vi "Get DBECU Reference.vi"(8 "error in (no error)":errorcluster, 10 "Alias":string, 11 "Device Item Ref in":T1 format="%.0x") -> (0 "error out":errorcluster, 1 "empty?":bool, 2 "XNET ECU":refnum<k21>, 3 "Device Item Ref out":T1 format="%.0x", 5 "XNET Cluster":refnum<k21>)   [LabVIEW 2018, in "CAN Gateway System Explorer.lvlib"]
uses:
  CAN Gateway System Explorer.lvlib
  <vilib>/NI Veristand/Custom Device API/Custom Device Item Ref.ctl
  Shared/Constants.vi
  <vilib>/NI Veristand/Custom Device API/Get Item Property (String).vi
  <resource>/objmgr/xnet.rc
  <vilib>/NI Veristand/Custom Device API/Custom Device API.lvlib
  Shared/CAN Gateway Shared.lvlib
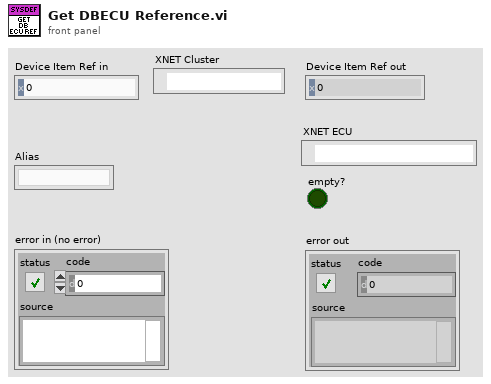
[diagram p1: front panel]
types:
  T1 = typedef "Custom Device API.lvlib/Custom Device Item Ref.ctl" = u64
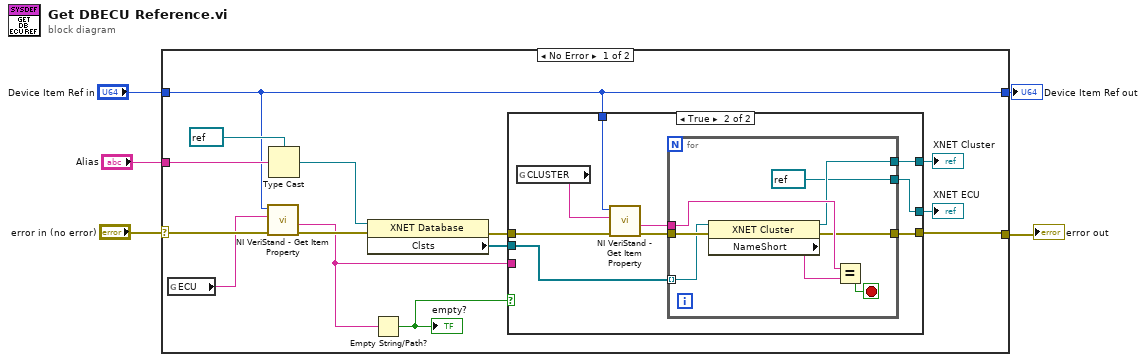
[diagram p0: block diagram]
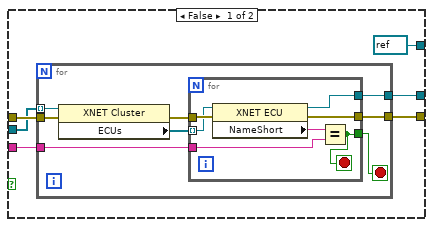
[diagram p2: hidden frame]
diagram:
  n1 = case shown="No Error" "error in (no error)" {
    selector: "error in (no error)" -> [w13 w59]
    tunnel: "Device Item Ref in" -> [w6 w58]
    tunnel: [w6 w58] -> w3
    tunnel: [w14 w59] -> w2
    tunnel: "Alias" -> [w19 _]
    frame No Error {
      n2 = global read "Constants.vi" "ECU"() -> (w12:string)
      n3 = call-poly <vilib>:"NI VeriStand - Get Item Property.vi"("error in (no error)"=w13, "Property Name"=w12, "Item Ref in"=w6) -> ("error out"=w11:errorcluster, "Value"=w9:string)  [unwired: 5 in, 2 out]
      n4 = Type Cast(type=refnum<k21> refnum ("XNET Database"), x=w19) -> (*(type *) &x=w17:refnum<k21>)
      n5 = property class="XNET Database"(reference=w17, error in=w11) -> (error out=w16:errorcluster, "Clsts"=w15:refnum<k21>[])  [unwired: 1 out]
      n6 = Empty String/Path?(string/path=w9) -> (empty?=w8:bool)
      "empty?" <- w8
      n7 = case shown="True" w8 {
        tunnel: w16 -> [w25 w48]
        tunnel: w15 -> [w24 w46]
        tunnel: [w23 w42] -> w14
        tunnel: [w22 w43] -> w10
        tunnel: w9 -> [w21 _]
        tunnel: [refnum<k21> refnum ("XNET Cluster") w44] -> w7
        tunnel: w6 -> [_ w41]
        frame False {
          n8 = for {
            tunnel: w25 -> [w33]
            tunnel: w24 -> [w32] mode=indexing
            tunnel: [w29] -> w23
            tunnel: w21 -> [w28]
            tunnel: [w27] -> w22
            stop <- w26 stop-if-true
            n9 = property class="XNET Cluster"(reference=w32, error in=w33) -> (error out=w30:errorcluster, "ECUs"=w31:refnum<k21>[])  [unwired: 1 out]
            n10 = for {
              tunnel: w31 -> [w39] mode=indexing
              tunnel: w30 -> [w40]
              tunnel: [w38] -> w29
              tunnel: w28 -> [w36]
              tunnel: [w35] -> w27
              tunnel: [w34] -> w26
              stop <- w34 stop-if-true
              n11 = property class="XNET ECU"(reference=w39, error in=w40) -> (reference out=w35:refnum<k21>, error out=w38:errorcluster, "NameShort"=w37:string)
              n12 = Equal?(x=w37, y=w36) -> (x = y?=w34:bool)
            }
          }
        }
        frame True {
          n13 = global read "Constants.vi" "CLUSTER"() -> (w49:string)
          n14 = call-poly <vilib>:"NI VeriStand - Get Item Property.vi"("error in (no error)"=w48, "Property Name"=w49, "Item Ref in"=w41) -> ("error out"=w47:errorcluster, "Value"=w45:string)  [unwired: 5 in, 2 out]
          n15 = for {
            tunnel: w47 -> [w57]
            tunnel: w46 -> [w56] mode=indexing
            tunnel: w45 -> [w54]
            tunnel: [w52] -> w44
            tunnel: [refnum<k21> refnum ("XNET ECU")] -> w43
            tunnel: [w50] -> w42
            stop <- w53 stop-if-true
            n16 = property class="XNET Cluster"(reference=w56, error in=w57) -> (reference out=w52:refnum<k21>, error out=w50:errorcluster, "NameShort"=w55:string)
            n17 = Equal?(x=w54, y=w55) -> (x = y?=w53:bool)
          }
        }
      }
      "XNET ECU" <- w10
      "XNET Cluster" <- w7
    }
    frame Error {
    }
  }
  "error out" <- w2
  "Device Item Ref out" <- w3
